vi "6-17 humidity.vi"() -> ()   [LabVIEW 2012]
uses:
  <vilib>/LabVIEW Hacker/LINX/Public/Peripherals/Analog/Analog Read 1 Chan.vi
  <vilib>/LabVIEW Hacker/LINX/LVH-LINX.lvlib
panel:
  in  "stop 2":bool
  out "humidity 2":dbl(graph)
  out "humidity  2":dbl
  in  "Serial Port":refnum<visa-resource-name>="COM4"
  in  "humidity":u8
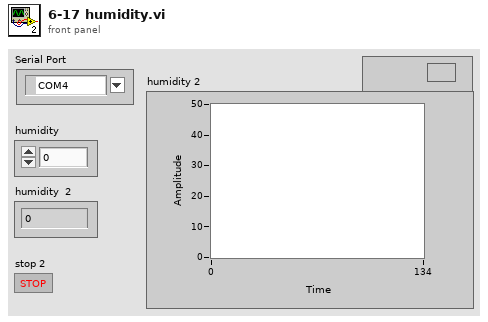
[diagram p1: front panel]
types:
  T1 = typedef "LVH-LINX.lvlib/LINX Ref.ctl" = cluster{"Platform":T2, "Interface":T3, "LINX Device Config":T4}
  T2 = typedef "LVH-LINX.lvlib/Platform.ctl" = enum16{"LINX", "myRIO"}
  T3 = typedef "LVH-LINX.lvlib/Interface.ctl" = enum16{"Serial", "TCP"}
  T4 = typedef "LVH-LINX.lvlib/Device.lvlib/LINX Device Config.ctl" = cluster{"Interface":T3, "COM Port":refnum<visa-resource-name>, "TCP Configuration":T5, "Device Family":T6, "Device ID":u8, "Device Name":string, "TCP Ref":refnum<k5>}
  T5 = typedef "LVH-LINX.lvlib/Device.lvlib/TCP Config.ctl" = cluster{"IP Address":string, "Port":u16}
  T6 = typedef "LVH-LINX.lvlib/Device Family.ctl" = enum8{"National Instruments", "Digilent", "Arduino"}
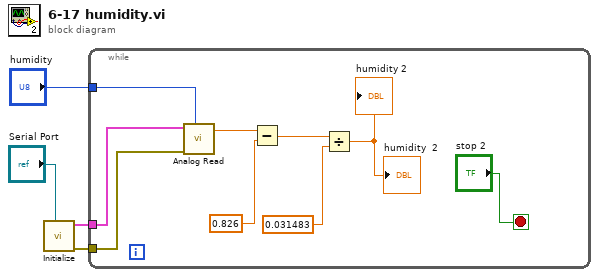
[diagram p0: block diagram]
diagram:
  n1 = call <vilib>:"Initialize.vi"("Serial Port"="Serial Port") -> ("Error Out"=w1:errorcluster, "LINX Ref"=w3:T1)  [unwired: 8 in, 1 out]
  n2 = while {
    tunnel: w3 -> [w12]
    tunnel: "humidity" -> [w13]
    tunnel: w1 -> [w11]
    stop <- "stop 2" stop-if-true
    n3 = call-poly <vilib>:"Analog Read.vi"("Analog Ref Override"=w13, "Error In"=w11, "LINX Resource"=w12) -> ("AI Value"=w7:dbl)  [unwired: 5 in, 3 out]
    n4 = Subtract(x=w7, y=0.826) -> (x-y=w9:dbl)
    n5 = Divide(x=w9, y=0.031483) -> (x/y=→"humidity  2" →"humidity 2":dbl)
  }
